vi "Exercicio2410.vi"() -> ()   [LabVIEW 2017]
panel:
  out "Sistema 2":bool
  out "Sistema 1":bool
  in  "Seleção do sistema para aquisição":bool
  out "Tempo decorrido (s)":dbl
  out "Corrente de saída do Sistema 2":dbl
  out "Corrente de saída do Sistema 1":dbl
  out "Sistema 2 (psi)":dbl(knob) scale=50.0..110.0
  out "Sistema 1 (psi)":dbl(knob) scale=0.0..60.0
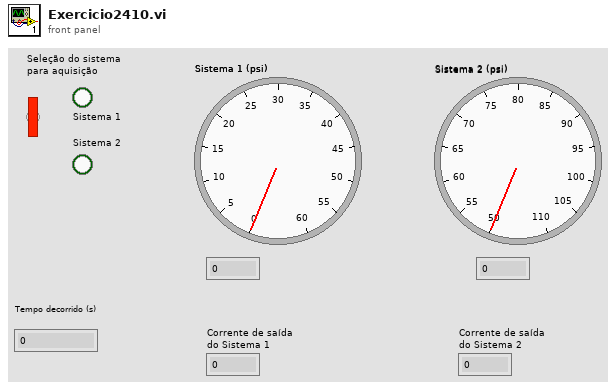
[diagram p1: front panel]
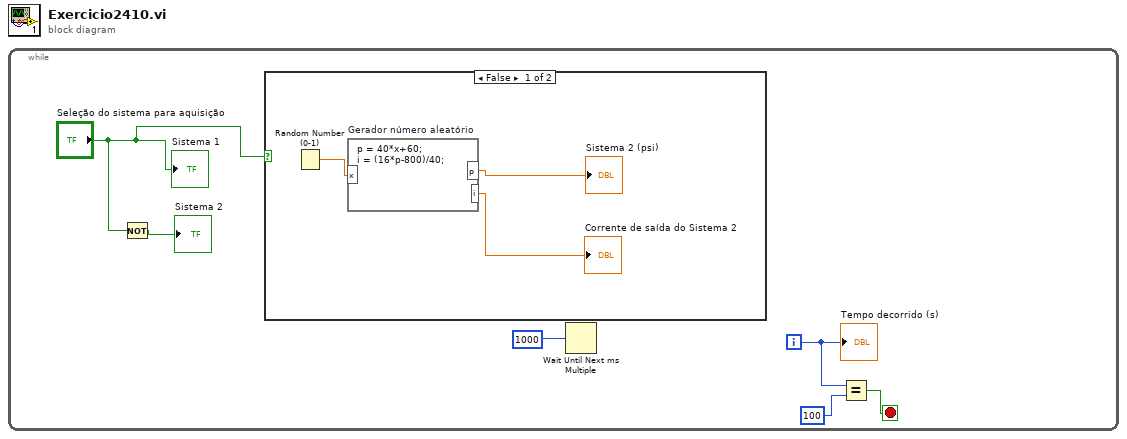
[diagram p0: block diagram]
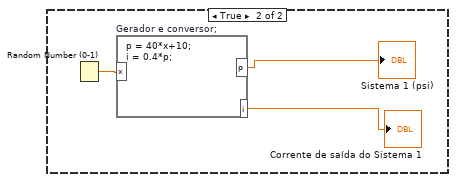
[diagram p2: hidden frame]
diagram:
  n1 = while {
    i -> [w2]
    stop <- w3 stop-if-true
    n2 = Not(x="Seleção do sistema para aquisição") -> (.not. x?=→"Sistema 2":bool)
    n3 = case shown="False" "Seleção do sistema para aquisição" {
      frame False {
        n4 = Random Number (0-1)() -> (number: 0 to 1=w9:dbl)
        n5 = formula code="p = 40*x+60;\ni = (16*p-800)/40;" "Gerador número aleatório"("x"=w9) -> ("p"=→"Sistema 2 (psi)":dbl, "i"=→"Corrente de saída do Sistema 2":dbl)
      }
      frame True {
        n6 = Random Number (0-1)() -> (number: 0 to 1=w12:dbl)
        n7 = formula code="p = 40*x+10;\ni = 0.4*p;" "Gerador e conversor;"("x"=w12) -> ("p"=→"Sistema 1 (psi)":dbl, "i"=→"Corrente de saída do Sistema 1":dbl)
      }
    }
    n8 = Wait Until Next ms Multiple(millisecond multiple=1000) -> ()  [unwired: 1 out]
    n9 = Equal?(x=w2, y=100) -> (x = y?=w3:bool)
    "Tempo decorrido (s)" <- w2
    "Sistema 1" <- "Seleção do sistema para aquisição"
  }
